vi "Teleop.vi"(10 "Match Info":T1={"Autonomous Elapsed Seconds"=0.0, "TeleOp Elapsed Seconds"=0.0, "Disabled Elapsed Seconds"=0.0, "Visited Autonomous"=FALSE, "Visited TeleOp"=FALSE, "Visited Disabled"=FALSE, "Autonomous Settings"={"Autonomous Style"=enum."Independent", "VI Refnum"=refnum}}, 11 "Call Context":T2) -> ()   [LabVIEW 2014]
doc: "This VI is called for each TeleOp packet received from the DS where the robot is not disabled. It is often used to read from the joysticks and update I/O or to update setpoints for timed control loops. It should complete and return within 20 milliseconds or it may miss DS packets."
uses:
  <vilib>/Rock Robotics/WPI/DriverStation/WPI_DriverStationDerivedRobotMode.ctl
  <vilib>/Rock Robotics/WPI/DriverStation/WPI_DriverStationMatch Info.ctl
  <vilib>/Rock Robotics/WPI/Joystick/WPI_JoystickGetSetRefNum.vi
  <vilib>/Rock Robotics/Network Tables/SD Write Boolean Array.vi
  <vilib>/Rock Robotics/Network Tables/SD Write Numeric Array.vi
  <vilib>/Rock Robotics/Network Tables/SD Read Boolean.vi
  <vilib>/Rock Robotics/Network Tables/SD Read Number.vi
  <vilib>/Rock Robotics/WPI/RobotDrive/WPI_RobotDriveGetSetRefNum.vi
  <vilib>/addons/control/pid/pid.llb/PID Advanced (DBL).vi
  <vilib>/Rock Robotics/WPI/RobotDrive/WPI_RobotDriveMecanumDrive_Cartesian.vi
  <vilib>/addons/control/pid/NI_PID_pid.lvlib
panel:
  in  "practice bot":bool=TRUE
  in  "stop motors":bool
  in  "set y":dbl format="%#_13g"
  in  "set x":dbl format="%#_13g"
  out "heading":i16
  out "pos y":i16
  out "pos x":i16
  out "distance":fxp<+/-,32,16>[](array[numeric])
  in  "test get data":bool=TRUE
  in  "test drive":bool
  out "Sample Slider 0":dbl(slide) scale=0.0..5.0
  out "Sample Boolean 1":bool
  out "Sample Boolean 0":bool
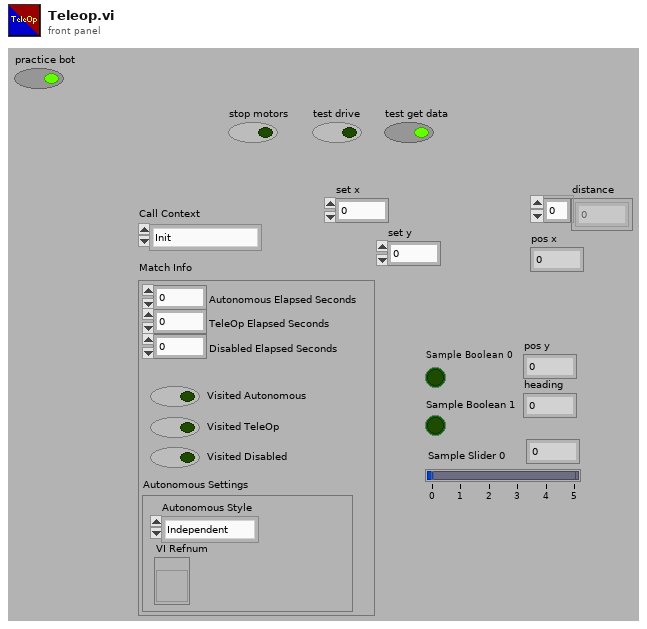
[diagram p1: front panel]
types:
  T1 = typedef "WPI_DriverStationMatch Info.ctl" = cluster{"Autonomous Elapsed Seconds":dbl, "TeleOp Elapsed Seconds":dbl, "Disabled Elapsed Seconds":dbl, "Visited Autonomous":bool, "Visited TeleOp":bool, "Visited Disabled":bool, "Autonomous Settings":cluster{"Autonomous Style":enum16{"Iterative", "Independent"}, "VI Refnum":refnum<vi>}}
  T2 = typedef "WPI_DriverStationDerivedRobotMode.ctl" = enum16{"Init", "Execute", "Stop"}
  T3 = cluster{"proportional gain (Kc)":dbl, "integral time (Ti, min)":dbl, "derivative time (Td, min)":dbl}
  T4 = typedef "WPI_JoystickDevRef.ctl" = cluster{"Device":T5}
  T5 = typedef "WPI_JoystickDeviceEnum.ctl" = enum16{"USB 0", "USB 1", "USB 2", "USB 3", "USB 4", "USB 5"}
  T6 = typedef "WPI_RobotDriveDevRef.ctl" = cluster{"DevStatus":errorcluster, "Motors[]":T7[], "Square Inputs":bool, "Max Output":dbl}
  T7 = typedef "WPI_MotorControlDeviceRef.ctl" = cluster{"DeviceStatus":errorcluster, "Type":T8, "PWM":cluster{"Controller":T9, "PWM Channel":T10, "DeadBand":T11}, "CAN":cluster{"Device Number":u8, "Control Mode":T12, "Semaphore":T13, "Max Vout":dbl, "TalonSRX Control Mode":T14}, "Invert":bool, "TransformRef":T15, "InvTransformRef":T15}
  T8 = typedef "WPI_MotorControlType.ctl" = enum16{"PWM", "CAN", "CANTalonSRX"}
  T9 = typedef "FPGA_TypedefDigitalModule.ctl" = enum16{"Controller 1"}
  T10 = typedef "FPGA_DIOPWMChannel.ctl" = enum8{"PWM 0", "PWM 1", "PWM 2", "PWM 3", "PWM 4", "PWM 5", "PWM 6", "PWM 7", "PWM 8", "PWM 9", "PWM MXP 0", "PWM MXP 1", "PWM MXP 2", "PWM MXP 3", "PWM MXP 4", "PWM MXP 5", "PWM MXP 6", "PWM MXP 7", "PWM MXP 8", "PWM MXP 9", "Invalid"}
  T11 = typedef "WPI_PWMDeadband.ctl" = cluster{"Name":string, "maxPositivePwm":i32, "minPositivePwm":i32, "centerPwm":i32, "maxNegativePwm":i32, "minNegativePwm":i32, "angularRange":u16}
  T12 = typedef "WPI_CANJaguar_ControlMode.ctl" = enum8{"Percent VBus", "Current", "Speed", "Position", "Voltage"}
  T13 = typedef "Semaphore RefNum" = refnum<k1>
  T14 = typedef "WPI_CANTalonSRX_APIControlMode.ctl" = enum8{"Percent VBus", "Speed", "Position", "Slave", "Unchanged / Invalid"}
  T15 = typedef "WPI_PWMTransform_ConPane.ctl" = refnum<vi>
  T16 = cluster{"Axes[0]":dbl, "Axes[1]":dbl, "Axes[2]":dbl, "Axes[3]":dbl, "Axes[4]":dbl, "Axes[5]":dbl, "Axes[6]":dbl, "Axes[7]":dbl, "Axes[8]":dbl}
  T17 = typedef "WPI_EncoderDevRef.ctl" = cluster{"DevStatus":errorcluster, "EncoderIndex":T18, "CounterIndex":T19, "DistancePerCount":dbl, "Decoding Type":T20}
  T18 = typedef "FPGA_EncoderIdx.ctl" = enum8{"Enc 0", "Enc 1", "Enc 2", "Enc 3", "Enc 4", "Enc 5", "Enc 6", "Enc 7", "Invalid"}
  T19 = typedef "FPGA_CounterCtrSystemIndex.ctl" = enum8{"Ctr 0", "Ctr 1", "Ctr 2", "Ctr 3", "Ctr 4", "Ctr 5", "Ctr 6", "Ctr 7", "Invalid"}
  T20 = typedef "WPI_EncoderType.ctl" = enum16{"1x", "2x", "4x"}
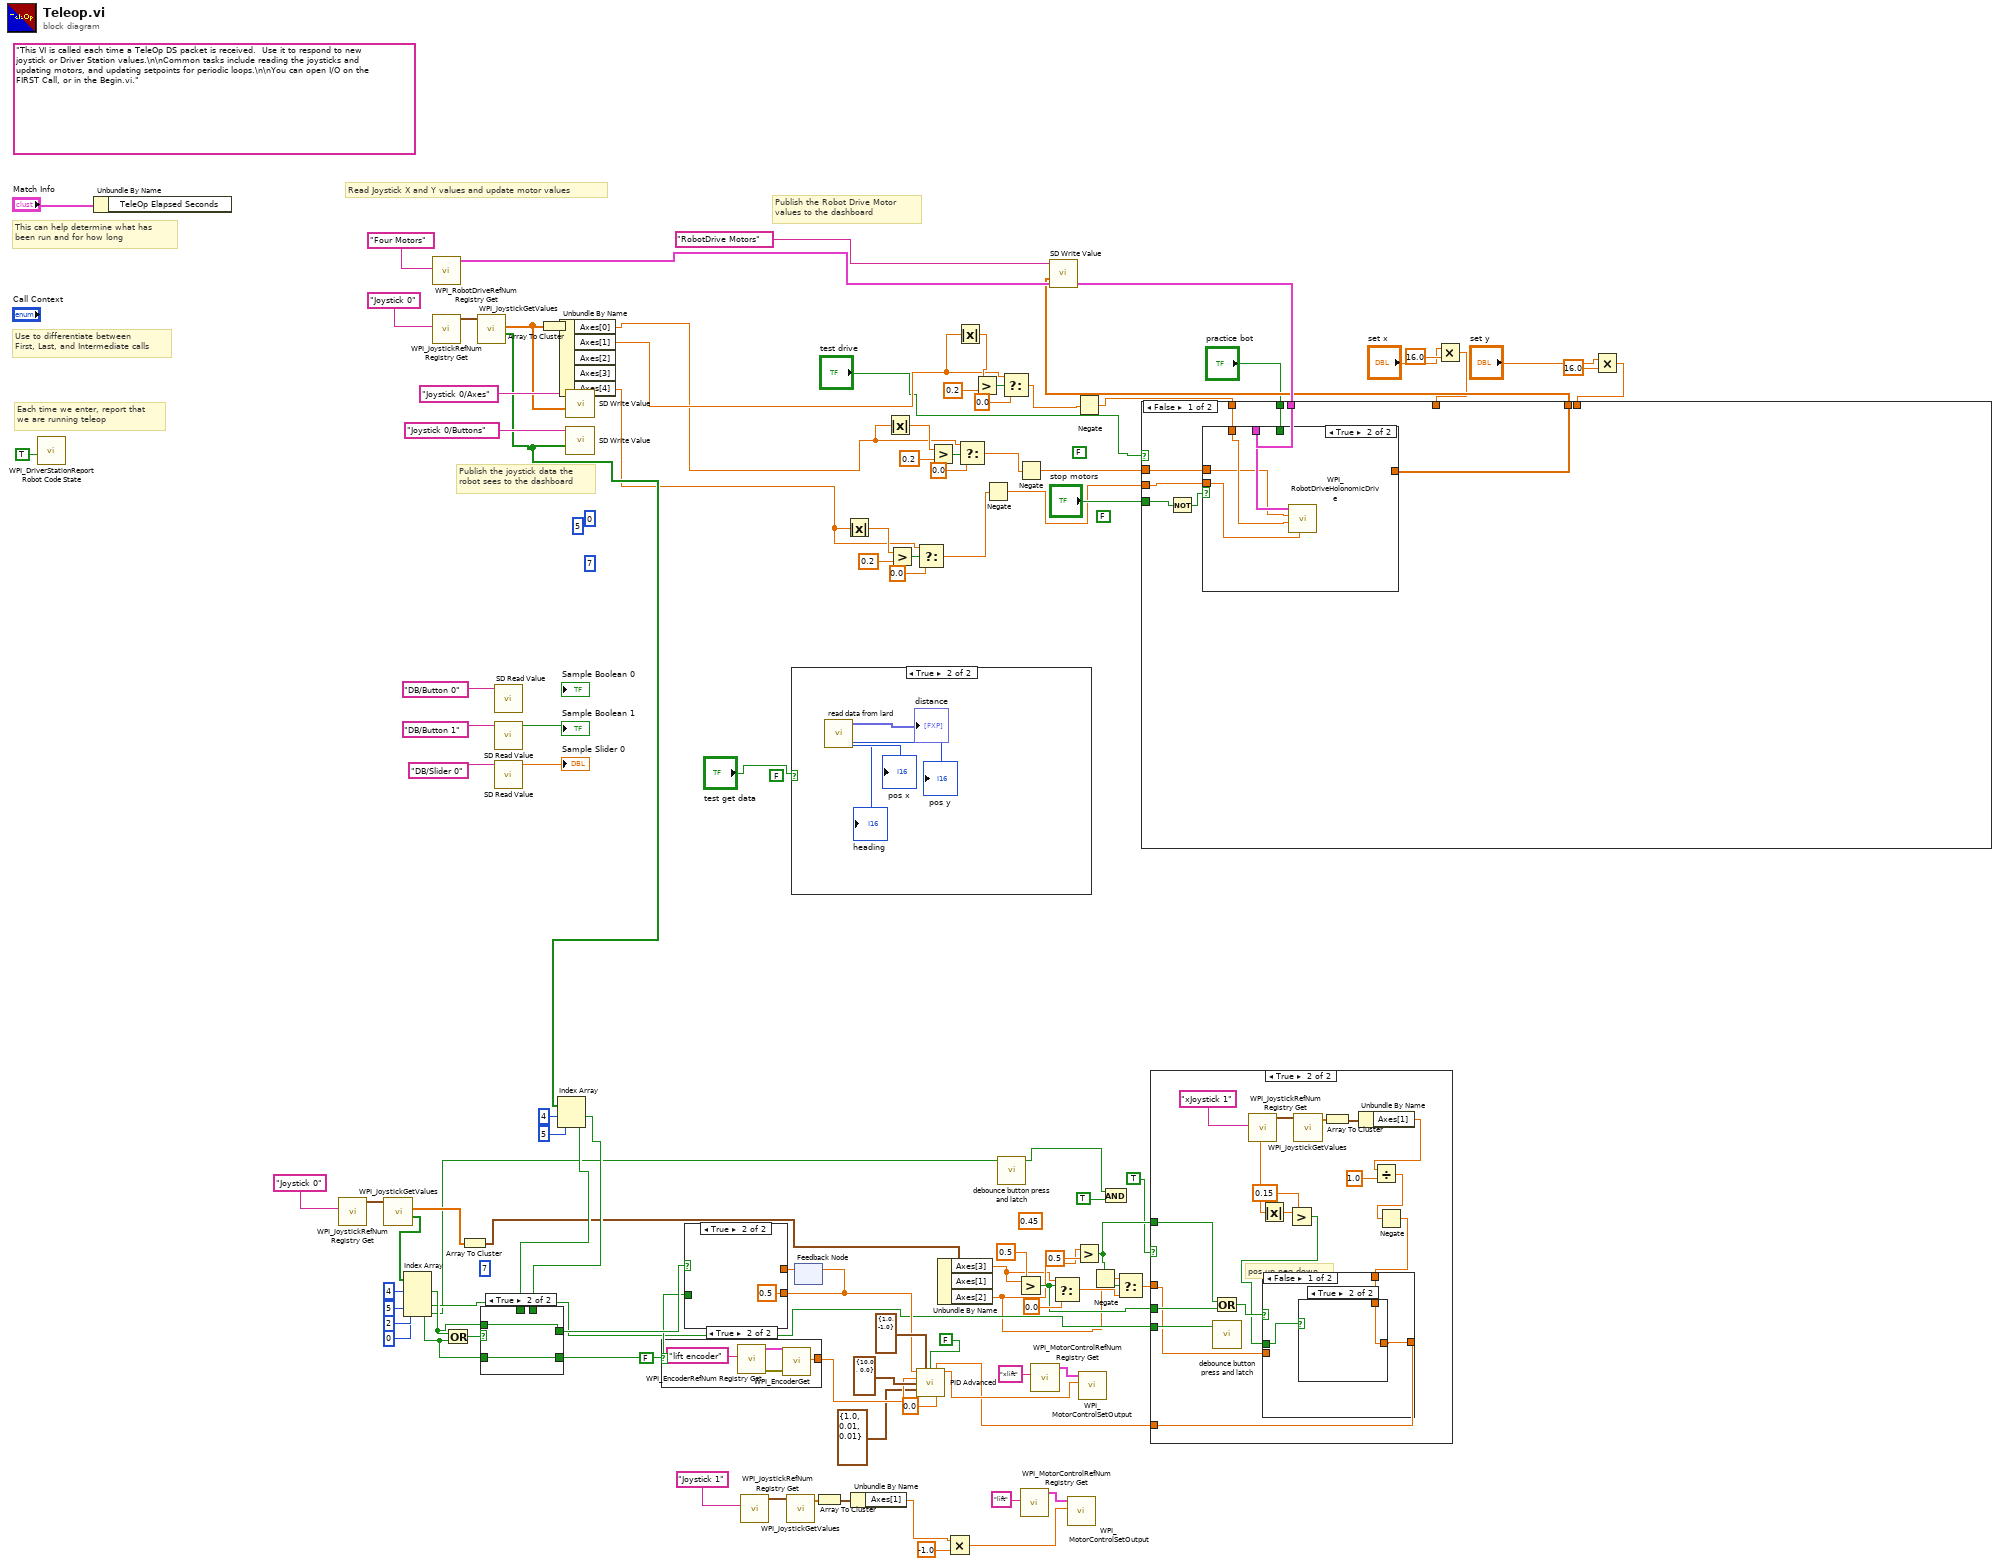
[diagram p0: block diagram]
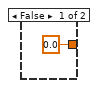
[diagram p4: hidden frame]
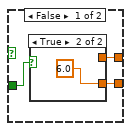
[diagram p7: hidden frame]
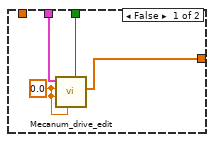
[diagram p10: hidden frame]
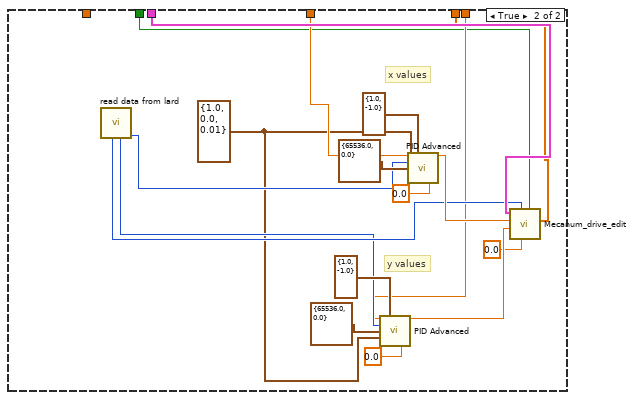
[diagram p11: hidden frame]
diagram:
  (unwired) FALSE
  (unwired) FALSE
  (unwired) FALSE
  (unwired) 0.45 ("t")
  (unwired) 7 ("index")
  (unwired) 7 ("index")
  (unwired) 5 ("index")
  (unwired) 0 ("index")
  (unwired) "This VI is called each time a TeleOp DS packet is received.  Use it to respond to new joystick or Driver Station values.\n\nCommon tasks include reading the joysticks and updating motors, and updating setpoints for periodic loops.\n\nYou can open I/O on the FIRST Call, or in the Begin.vi."
  # "Publish the Robot Drive Motor\nvalues to the dashboard"
  # "Publish the joystick data the\nrobot sees to the dashboard"
  # "Each time we enter, report that\nwe are running teleop"
  # "Use to differentiate between\nFirst, Last, and Intermediate calls"
  # "This can help determine what has\nbeen run and for how long"
  # "Read Joystick X and Y values and update motor values"
  n1 = call <vilib>:"WPI_DriverStationReport Robot Code State.vi"("TeleOp"=TRUE ("Autonomous")) -> ()  [unwired: 10 in, 1 out]
  n2 = Unbundle By Name("Match Info") -> ()  [unwired: 1 out]
  n3 = call <vilib>:"WPI_JoystickRefNum Registry Get.vi"("refnum name"="Joystick 0") -> ("JoystickDevRef"=w68:T4)  [unwired: 1 in, 9 out]
  n4 = call <vilib>:"WPI_JoystickGetValues.vi"("JoystickDevRef"=w68) -> ("Buttons"=w64:bool[], "Axes"=w57:dbl[])  [unwired: 6 in, 3 out]
  n5 = Index Array(array=w64, index #1=4 ("index"), index #2=5 ("index"), index #3=2 ("index"), index #4=0 ("index")) -> (element #1=w62:bool, element #2=w63:bool, element #3=w39:bool, element #4=w30:bool)
  n6 = call <vilib>:"WPI_RobotDriveRefNum Registry Get.vi"("refnum name"="Four Motors") -> ("RobotDriveDevRef"=w89:T6)  [unwired: 1 in, 9 out]
  n7 = call <vilib>:"WPI_JoystickRefNum Registry Get.vi"("refnum name"="Joystick 0") -> ("JoystickDevRef"=w101:T4)  [unwired: 1 in, 9 out]
  n8 = Or(x=w62, y=w63) -> (x .or. y?=w67:bool)
  n9 = Array To Cluster(array=w57) -> (cluster=w56:T16)
  n10 = call <vilib>:"WPI_JoystickGetValues.vi"("JoystickDevRef"=w101) -> ("Buttons"=w70:bool[], "Axes"=w91:dbl[])  [unwired: 6 in, 3 out]
  n11 = call-poly <vilib>:"SD Read Value.vi"("Name"="DB/Button 0" ("refnum name")) -> ()  [unwired: 8 in, 3 out]
  n12 = call-poly <vilib>:"SD Read Value.vi"("Name"="DB/Button 1" ("refnum name")) -> ("Boolean"=→"Sample Boolean 1":bool)  [unwired: 8 in, 2 out]
  n13 = call-poly <vilib>:"SD Read Value.vi"("Name"="DB/Slider 0" ("refnum name")) -> ("Numeric"=→"Sample Slider 0":dbl)  [unwired: 8 in, 2 out]
  n14 = Array To Cluster(array=w91) -> (cluster=w90:T16)
  n15 = Index Array(array=w70, index #1=4 ("index"), index #2=5 ("index")) -> (element #1=w59:bool, element #2=w58:bool)
  n16 = case shown="True" w67 {
    tunnel: [w105 w108] -> w60
    tunnel: w63 -> [_ w108]
    tunnel: [w106 w107] -> w61
    tunnel: w62 -> [_ w107]
    tunnel: w59 -> [w106 _]
    tunnel: w58 -> [w105 _]
    frame False {
    }
    frame True {
    }
  }
  n17 = Unbundle By Name(w90) -> ("Axes[0]"=w40:dbl, "Axes[1]"=w42:dbl, "Axes[4]"=w21:dbl)  [unwired: 2 out]
  n18 = call-poly <vilib>:"SD Write Value.vi"("Numeric Array"=w91, "Name"="Joystick 0/Axes") -> ()  [unwired: 8 in, 2 out]
  n19 = call-poly <vilib>:"SD Write Value.vi"("Boolean Array"=w70, "Name"="Joystick 0/Buttons") -> ()  [unwired: 8 in, 2 out]
  n20 = case shown="True" FALSE {
    tunnel: [_ w110] -> w76
    frame False {
    }
    frame True {
      n21 = call <vilib>:"WPI_EncoderRefNum Registry Get.vi"("refnum name"="lift encoder") -> ("error out"=w112:errorcluster, "EncoderDevRef"=w111:T17)  [unwired: 9 in]
      n22 = call <vilib>:"WPI_EncoderGet.vi"("error in (no error)"=w112, "EncoderDevRef"=w111) -> ("Distance"=w110:dbl)  [unwired: 4 in, 5 out]
    }
  }
  n23 = call <vilib>:"WPI_JoystickRefNum Registry Get.vi"("refnum name"="Joystick 1") -> ("JoystickDevRef"=w16:T4)  [unwired: 1 in, 9 out]
  n24 = call <vilib>:"WPI_JoystickGetValues.vi"("JoystickDevRef"=w16) -> ("Axes"=w15:dbl[])  [unwired: 6 in, 4 out]
  n25 = case shown="True" "test get data" {
    frame False {
    }
    frame True {
      n26 = call "read data from lard.vi"() -> ("pos x"=→"pos x":i16, "distance"=→"distance":fxp<+/-,32,16>[], "pos y"=→"pos y":i16, "heading"=→"heading":i16)  [unwired: 8 in]
    }
  }
  n27 = feedback #1() -> (w71:dbl)  [unwired: 1 in]
  n28 = case shown="True" w61 {
    tunnel: w60 -> [w119 _]
    tunnel: [w118 0.5 ("Output")] -> w72
    tunnel: w71 -> [w117 _]
    frame False {
      n29 = case shown="True" w119 {
        tunnel: [w120 6.0 ("Output")] -> w118
        tunnel: w117 -> [w120 _]
        frame False {
        }
        frame True {
        }
      }
    }
    frame True {
    }
  }
  n30 = feedback-in #1(w72) -> ()
  n31 = Array To Cluster(array=w15) -> (cluster=w14:T16)
  n32 = Absolute Value(x=w21) -> (abs(x)=w22:dbl)
  n33 = Unbundle By Name(w14) -> ("Axes[1]"=w13:dbl)
  n34 = Absolute Value(x=w40) -> (abs(x)=w41:dbl)
  n35 = Greater?(x=w22, y=0.2) -> (0:w25:bool)
  n36 = Select(t=w21, s=w25, f=0.0) -> (s? t:f=w2:dbl)
  n37 = Greater?(x=w41, y=0.2) -> (0:w47:bool)
  n38 = Unbundle By Name(w56) -> ("Axes[3]"=w8:dbl, "Axes[2]"=w9:dbl)  [unwired: 1 out]
  n39 = Multiply(x=w13, y=-1.0) -> (x*y=w12:dbl)
  n40 = Absolute Value(x=w42) -> (abs(x)=w43:dbl)
  n41 = Select(t=w40, s=w47, f=0.0) -> (s? t:f=w6:dbl)
  n42 = Greater?(x=w43, y=0.2) -> (0:w49:bool)
  n43 = Negate(x=w2) -> (-x=w1:dbl)
  n44 = call "debounce button press and latch.vi"("Boolean"=w30) -> ("Boolean 2"=w33:bool)  [unwired: 10 in]
  n45 = Select(t=w42, s=w49, f=0.0) -> (s? t:f=w4:dbl)
  n46 = Greater?(x=w8, y=0.5) -> (0:w38:bool)
  n47 = Negate(x=w6) -> (-x=w5:dbl)
  n48 = call <vilib>:"WPI_MotorControlRefNum Registry Get.vi"("refnum name"="lift") -> ("MotorControlDevRef"=w18:T7)  [unwired: 9 in, 1 out]
  n49 = call <vilib>:"WPI_MotorControlRefNum Registry Get.vi"("refnum name"="xlift") -> ("MotorControlDevRef"=w73:T7)  [unwired: 9 in, 1 out]
  n50 = Select(t=w8, s=w38, f=0.0) -> (s? t:f=w36:dbl)
  n51 = call <vilib>:"WPI_MotorControlSetOutput.vi"("Output"=w12, "MotorControlDevRef"=w18) -> ()  [unwired: 7 in, 3 out]
  n52 = Negate(x=w4) -> (-x=w3:dbl)
  n53 = Greater?(x=w9, y=0.5) -> (0:w35:bool)
  n54 = Negate(x=w9) -> (-x=w10:dbl)
  n55 = And(x=w33, y=TRUE) -> ()  [unwired: 1 out]
  n56 = Select(t=w10, s=w35, f=w36) -> (s? t:f=w34:dbl)
  n57 = case shown="True" TRUE {
    tunnel: w39 -> [_ w140]
    tunnel: w38 -> [_ w134]
    tunnel: [w123 w132] -> w37
    tunnel: w35 -> [_ w128]
    tunnel: w34 -> [w123 w127]
    frame False {
    }
    frame True {
      # "pos up neg down"
      n58 = Or(x=w128, y=w134) -> (x .or. y?=w135:bool)
      n59 = call "debounce button press and latch.vi"("Boolean"=w140) -> ()  [unwired: 10 in, 1 out]
      n60 = call <vilib>:"WPI_JoystickRefNum Registry Get.vi"("refnum name"="xJoystick 1") -> ("JoystickDevRef"=w138:T4)  [unwired: 1 in, 9 out]
      n61 = call <vilib>:"WPI_JoystickGetValues.vi"("JoystickDevRef"=w138) -> ("Axes"=w137:dbl[])  [unwired: 6 in, 4 out]
      n62 = Array To Cluster(array=w137) -> (cluster=w136:T16)
      n63 = Unbundle By Name(w136) -> ("Axes[1]"=w126:dbl)
      n64 = Absolute Value(x=w126) -> (abs(x)=w131:dbl)
      n65 = Greater?(x=w131, y=0.15) -> (0:w129:bool)
      n66 = Divide(x=w126, y=1.0) -> (x/y=w124:dbl)
      n67 = Negate(x=w124) -> (-x=w133:dbl)
      n68 = case shown="False" w135 {
        tunnel: w129 -> [w143 _]
        tunnel: [w142 w146] -> w132
        tunnel: w127 -> [_ w146]
        tunnel: w133 -> [w141 _]
        frame False {
          n69 = case shown="True" w143 {
            tunnel: [0.0 w145] -> w142
            tunnel: w141 -> [_ w145]
            frame False {
            }
            frame True {
            }
          }
        }
        frame True {
        }
      }
    }
  }
  n70 = call-poly <vilib>:"PID Advanced.vi"("setpoint"=w72, "output range"=cluster{"output high":dbl, "output low":dbl} {"output high"=1.0, "output low"=-1.0}, "auto? (T)"=FALSE, "manual control"=w37, "process variable"=w76, "setpoint range"=cluster{"setpoint high":dbl, "setpoint low":dbl} {"setpoint high"=10.0, "setpoint low"=0.0}, "PID gains"=T3 {"proportional gain (Kc)"=1.0, "integral time (Ti, min)"=0.01, "derivative time (Td, min)"=0.01}, "linearity"=0.0) -> ("output"=w50:dbl)  [unwired: 6 in, 1 out]
  n71 = call <vilib>:"WPI_MotorControlSetOutput.vi"("Output"=w50, "MotorControlDevRef"=w73) -> ()  [unwired: 7 in, 3 out]
  n72 = Multiply(x="set x", y=16.0) -> (x*y=w83:dbl)
  n73 = Multiply(x="set y", y=16.0) -> (x*y=w82:dbl)
  n74 = case shown="False" "test drive" {
    tunnel: w89 -> [w154 w171]
    tunnel: w3 -> [w153 _]
    tunnel: w5 -> [w152 _]
    tunnel: [w151 w164] -> w88
    tunnel: w83 -> [_ w167]
    tunnel: w82 -> [_ w166]
    tunnel: "stop motors" -> [w149 _]
    tunnel: "practice bot" -> [w148 w163]
    tunnel: w1 -> [w147 _]
    frame False {
      n75 = Not(x=w149) -> (.not. x?=w150:bool)
      n76 = case shown="True" w150 {
        tunnel: w154 -> [w158 w162]
        tunnel: w153 -> [_ w161]
        tunnel: w152 -> [_ w160]
        tunnel: [w156 _] -> w151
        tunnel: w148 -> [w155 _]
        tunnel: w147 -> [_ w159]
        frame False {
          w157 = 0.0 ("X")
          n77 = call "Mecanum_drive_edit.vi"("practice bot"=w155, "Rotation"=w157, "Y"=w157, "X"=w157, "RobotDriveDevRef"=w158) -> ("Motor Values"=w156:dbl[])  [unwired: 4 in, 2 out]
        }
        frame True {
          n78 = call-poly <vilib>:"WPI_RobotDriveHolonomicDrive.vi"("Rotation"=w159, "Y"=w161, "X"=w160, "RobotDriveDevRef"=w162) -> ()  [unwired: 5 in, 3 out]
        }
      }
    }
    frame True {
      w165 = T3 {"proportional gain (Kc)"=1.0, "integral time (Ti, min)"=0.0, "derivative time (Td, min)"=0.01} ("PID gains")
      # "y values"
      # "x values"
      n79 = call "read data from lard.vi"() -> ("pos x"=w169:i16, "pos y"=w168:i16, "heading"=w170:i16)  [unwired: 8 in, 1 out]
      n80 = call-poly <vilib>:"PID Advanced.vi"("setpoint"=w166, "output range"=cluster{"output high":dbl, "output low":dbl} {"output high"=1.0, "output low"=-1.0}, "process variable"=w168, "setpoint range"=cluster{"setpoint high":dbl, "setpoint low":dbl} {"setpoint high"=65536.0, "setpoint low"=0.0}, "PID gains"=w165, "linearity"=0.0) -> ("output"=w173:dbl)  [unwired: 8 in, 1 out]
      n81 = call-poly <vilib>:"PID Advanced.vi"("setpoint"=w167, "output range"=cluster{"output high":dbl, "output low":dbl} {"output high"=1.0, "output low"=-1.0}, "process variable"=w169, "setpoint range"=cluster{"setpoint high":dbl, "setpoint low":dbl} {"setpoint high"=65536.0, "setpoint low"=0.0}, "PID gains"=w165, "linearity"=0.0) -> ("output"=w174:dbl)  [unwired: 8 in, 1 out]
      n82 = call "Mecanum_drive_edit.vi"("practice bot"=w163, "Rotation"=0.0, "Gyro Angle"=w170, "Y"=w173, "X"=w174, "RobotDriveDevRef"=w171) -> ("Motor Values"=w164:dbl[])  [unwired: 3 in, 2 out]
    }
  }
  n83 = call-poly <vilib>:"SD Write Value.vi"("Numeric Array"=w88, "Name"="RobotDrive Motors") -> ()  [unwired: 8 in, 2 out]
